vi "Query with Scalar Integer Result.vi"(8 "error in (no error)":errorcluster, 10 "Query string":string, 11 "mysql in":refnum<class "mysql.lvclass">) -> (0 "error out":errorcluster, 2 "Result":i32, 3 "mysql out":refnum<class "mysql.lvclass">)   [LabVIEW 2020, in "mysql.lvlib" / "mysql.lvclass"]
uses:
  mysql.lvclass
  efc009f7-6f9b-4833-9fcc-8bf45dc70998.vi
  efc009f7-6f9b-4833-9fcc-8bf45dc70998.vi/094420c8-9f98-4731-a090-4e87c68797ae.vi
  private/Mysql command.vi
  private/Mysql data reader scalar integer.vi
  private/ping connection and reopen if needed.vi
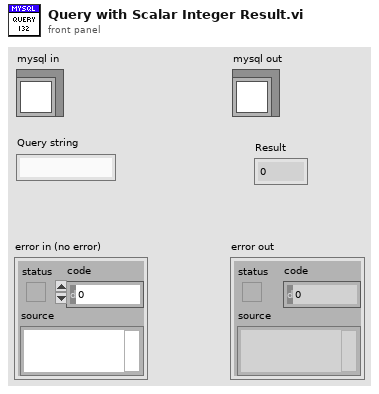
[diagram p1: front panel]
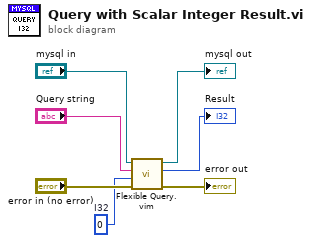
[diagram p0: block diagram]
diagram:
  w4 = 0  # I32
  n1 = call "Flexible Query.vim"("error in (no error)"="error in (no error)", "Type in"=w4, "Query string"="Query string", "mysql in"="mysql in") -> ("error out"=→"error out":errorcluster, "Result"=→"Result":i32, "mysql out"=→"mysql out":refnum<class "mysql.lvclass">)  [unwired: 5 in]
